vi "Read Joystick.vi"(8 "Joystick Deadbanded Value (default of 0.1)":dbl, 11 "Joystick L 1 DevRef":T1) -> (1 "Joystick R 2 X Axis":dbl, 2 "Joystick L 1 Y Axis":dbl, 3 "Joystick L 1 X Axis":dbl)   [LabVIEW 2014]
uses:
  <vilib>/Rock Robotics/WPI/Joystick/WPI_JoystickDevRef.ctl
  <vilib>/Rock Robotics/WPI/Joystick/WPI_JoystickDeviceEnum.ctl
  Global Variables.vi
  <vilib>/Rock Robotics/WPI/Joystick/WPI_JoystickGetSetRefNum.vi
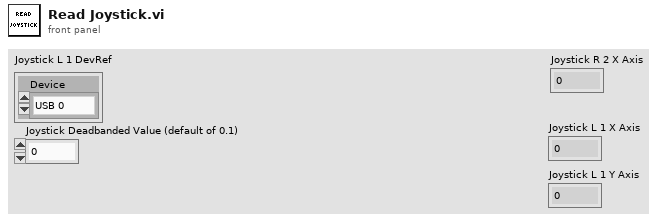
[diagram p1: front panel]
types:
  T1 = typedef "WPI_JoystickDevRef.ctl" = cluster{"Device":T2}
  T2 = typedef "WPI_JoystickDeviceEnum.ctl" = enum16{"USB 0", "USB 1", "USB 2", "USB 3", "USB 4", "USB 5"}
  T3 = cluster{"Axes[0]":dbl, "Axes[1]":dbl, "Axes[2]":dbl, "Axes[3]":dbl, "Axes[4]":dbl, "Axes[5]":dbl, "Axes[6]":dbl, "Axes[7]":dbl, "Axes[8]":dbl}
  T4 = cluster{"Buttons[0]":bool, "Buttons[1]":bool, "Buttons[2]":bool, "Buttons[3]":bool, "Buttons[4]":bool, "Buttons[5]":bool, "Buttons[6]":bool, "Buttons[7]":bool, "Buttons[8]":bool}
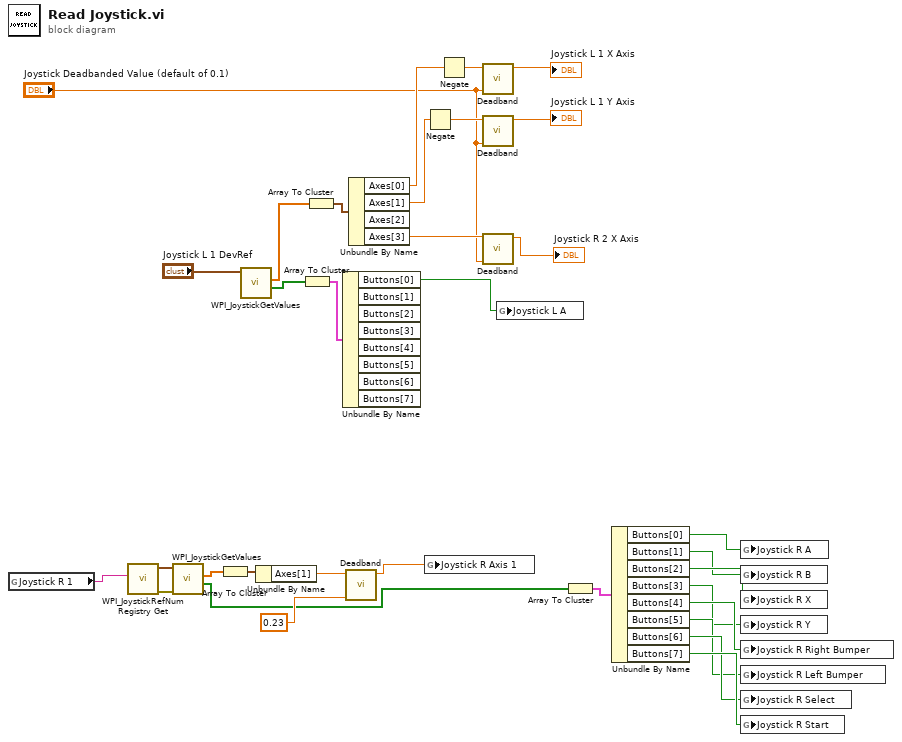
[diagram p0: block diagram]
diagram:
  n1 = global read "Global Variables.vi" "Joystick R 1"() -> (w17:string)
  n2 = call <vilib>:"WPI_JoystickRefNum Registry Get.vi"("refnum name"=w17) -> ("error out"=w16:errorcluster, "JoystickDevRef"=w15:T1)  [unwired: 9 in]
  n3 = call <vilib>:"WPI_JoystickGetValues.vi"("error in (no error)"=w16, "JoystickDevRef"=w15) -> ("Buttons"=w3:bool[], "Axes"=w18:dbl[])  [unwired: 5 in, 3 out]
  n4 = Array To Cluster(array=w18) -> (cluster=w19:T3)
  n5 = call <vilib>:"WPI_JoystickGetValues.vi"("JoystickDevRef"="Joystick L 1 DevRef") -> ("Buttons"=w30:bool[], "Axes"=w32:dbl[])  [unwired: 6 in, 3 out]
  n6 = Unbundle By Name(w19) -> ("Axes[1]"=w13:dbl)
  n7 = Array To Cluster(array=w30) -> (cluster=w29:T4)
  n8 = Array To Cluster(array=w32) -> (cluster=w31:T3)
  n9 = Unbundle By Name(w29) -> ("Buttons[0]"=w1:bool)  [unwired: 7 out]
  n10 = call "Deadband.vi"("Value to Deadband (default of 0.1)"=0.23, "Value"=w13) -> ("Deadbanded Value"=w12:dbl)  [unwired: 9 in]
  n11 = Unbundle By Name(w31) -> ("Axes[0]"=w28:dbl, "Axes[1]"=w23:dbl, "Axes[3]"=w22:dbl)  [unwired: 1 out]
  n12 = Negate(x=w23) -> (-x=w24:dbl)
  n13 = global write "Global Variables.vi" "Joystick R Axis 1"(w12) -> ()
  n14 = Negate(x=w28) -> (-x=w27:dbl)
  n15 = call "Deadband.vi"("Value to Deadband (default of 0.1)"="Joystick Deadbanded Value (default of 0.1)", "Value"=w27) -> ("Deadbanded Value"=→"Joystick L 1 X Axis":dbl)  [unwired: 9 in]
  n16 = call "Deadband.vi"("Value to Deadband (default of 0.1)"="Joystick Deadbanded Value (default of 0.1)", "Value"=w24) -> ("Deadbanded Value"=→"Joystick L 1 Y Axis":dbl)  [unwired: 9 in]
  n17 = call "Deadband.vi"("Value to Deadband (default of 0.1)"="Joystick Deadbanded Value (default of 0.1)", "Value"=w22) -> ("Deadbanded Value"=→"Joystick R 2 X Axis":dbl)  [unwired: 9 in]
  n18 = global write "Global Variables.vi" "Joystick L A"(w1) -> ()
  n19 = Array To Cluster(array=w3) -> (cluster=w4:T4)
  n20 = Unbundle By Name(w4) -> ("Buttons[0]"=w2:bool, "Buttons[1]"=w5:bool, "Buttons[2]"=w6:bool, "Buttons[3]"=w7:bool, "Buttons[4]"=w8:bool, "Buttons[5]"=w9:bool, "Buttons[6]"=w10:bool, "Buttons[7]"=w11:bool)
  n21 = global write "Global Variables.vi" "Joystick R A"(w2) -> ()
  n22 = global write "Global Variables.vi" "Joystick R B"(w5) -> ()
  n23 = global write "Global Variables.vi" "Joystick R X"(w6) -> ()
  n24 = global write "Global Variables.vi" "Joystick R Y"(w7) -> ()
  n25 = global write "Global Variables.vi" "Joystick R Right Bumper"(w8) -> ()
  n26 = global write "Global Variables.vi" "Joystick R Left Bumper"(w9) -> ()
  n27 = global write "Global Variables.vi" "Joystick R Select"(w10) -> ()
  n28 = global write "Global Variables.vi" "Joystick R Start"(w11) -> ()
